vi "DB-检查连接状态.vi"(8 "error in (no error)":errorcluster, 11 "数据库引用":T1) -> (0 "error out":errorcluster, 2 "连接正常?":bool, 3 "数据库连接引用out":T1)   [LabVIEW 2017]
uses:
  <vilib>/addons/database/Connection.llb/Conn ObjectReference.ctl
  <vilib>/addons/database/NI_Database_API.lvlib
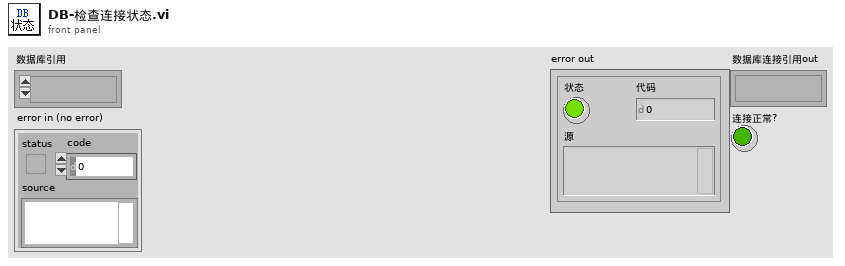
[diagram p1: front panel]
types:
  T1 = typedef "NI_Database_API.lvlib/Conn ObjectReference.ctl" = refnum<k1>
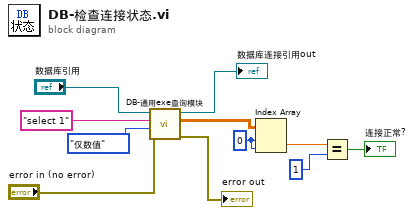
[diagram p0: block diagram]
diagram:
  w4 = 0 ("索引 (行)")
  n1 = call "DB-通用exe查询模块.vi"("error in (no error)"="error in (no error)", "解析模式"=enum16{"仅数值", "仅字符串", "数值与字符串"}."仅数值", "SQL query"="select 1", "数据库连接引用"="数据库引用") -> ("error out"=→"error out":errorcluster, "数值数据"=w6:dbl[][], "数据库连接引用out"=→"数据库连接引用out":T1)  [unwired: 3 in, 2 out]
  n2 = Index Array(array=w6, index (row)=w4, index (col)=w4) -> (element=w3:dbl)
  n3 = Equal?(x=w3, y=1 ("索引 (行)")) -> (x = y?=→"连接正常?":bool)
